vi "习题4.5.vi"() -> ()   [LabVIEW 2017]
panel:
  out "output":dbl
  in  "value":dbl
  out "count":dbl
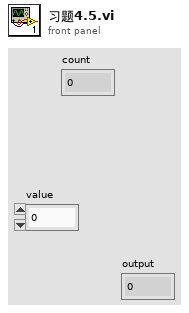
[diagram p1: front panel]
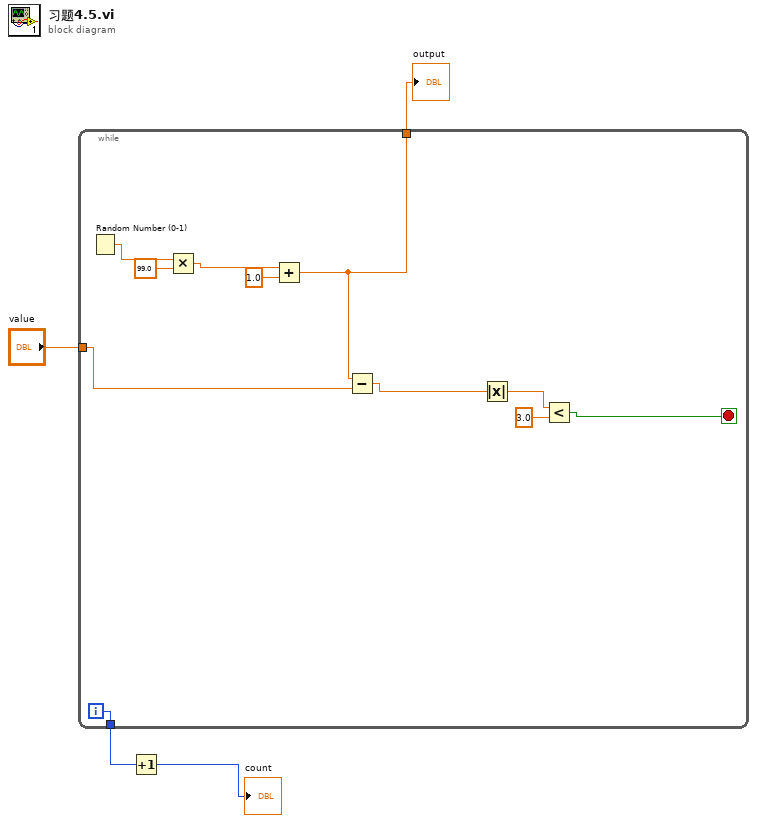
[diagram p0: block diagram]
diagram:
  n1 = while {
    tunnel: "value" -> [w9]
    tunnel: [w11] -> w2
    tunnel: [w10] -> w3
    i -> [w11]
    stop <- w5 stop-if-true
    n2 = Random Number (0-1)() -> (number: 0 to 1=w15:dbl)
    n3 = Multiply(x=w15, y=99.0) -> (x*y=w13:dbl)
    n4 = Add(x=w13, y=1.0) -> (x+y=w10:dbl)
    n5 = Subtract(x=w10, y=w9) -> (x-y=w8:dbl)
    n6 = Absolute Value(x=w8) -> (abs(x)=w7:dbl)
    n7 = Less?(x=w7, y=3.0) -> (x < y?=w5:bool)
  }
  "output" <- w3
  n8 = Increment(x=w2) -> (x+1=→"count":i32)
